vi "Overview of Qs.vi"() -> ()   [LabVIEW 2021, in "Qs.lvlib"]
uses:
  Qs.lvlib
panel:
  in  "Numeric Control":i32
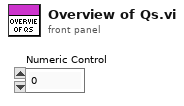
[diagram p1: front panel]
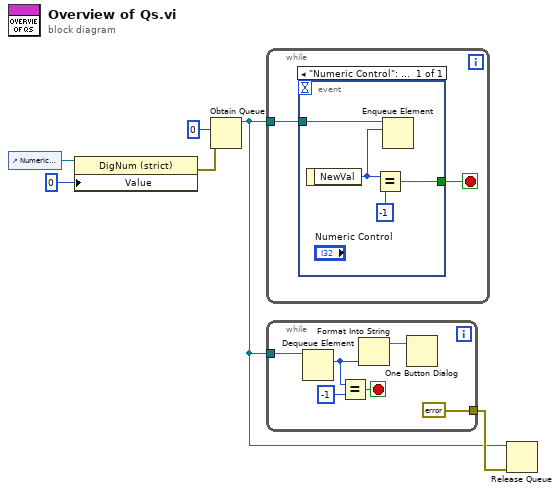
[diagram p0: block diagram]
diagram:
  n1 = control-ref of="Numeric Control"() -> (w6:refnum<vi>)
  n2 = property class="DigNum (strict)"(reference=w6, "Value"=0) -> (error out=w5:errorcluster)  [unwired: 1 in, 1 out]
  n3 = Obtain Queue(element data type=0 ("Value"), error in (no error)=w5) -> (queue out=w1:refnum<queue>)  [unwired: 3 in, 2 out]
  n4 = while {
    tunnel: w1 -> [w7]
    stop <- w8 stop-if-true
    n5 = event shown="[0] \"Numeric Control\": Value Change" {
      selector: _ -> [_]
      dyn-events: _ -> [_]
      timeout: _ -> [_]
      tunnel: w7 -> [w9]
      tunnel: [w11] -> w8
      event "Numeric Control": Value Change {
        n6 = event-data() -> ("NewVal"=w10:i32)  [unwired: 1 in]
        n7 = Equal?(x=w10, y=-1) -> (x = y?=w11:bool)
        n8 = Enqueue Element(queue=w9, element=w10) -> ()  [unwired: 2 in, 3 out]
      }
    }
  }
  n9 = while {
    tunnel: w1 -> [w15]
    tunnel: [errorcluster {"status"=FALSE, "code"=0, "source"=""} ("error in (no error)")] -> w3
    stop <- w18 stop-if-true
    n10 = Dequeue Element(queue=w15) -> (element=w13:i32)  [unwired: 2 in, 3 out]
    n11 = Equal?(x=w13, y=-1) -> (x = y?=w18:bool)
    n12 = Format Into String(w13) -> (resulting string=w14:string)  [unwired: 3 in, 1 out]
    n13 = One Button Dialog(message=w14) -> ()  [unwired: 1 in, 1 out]
  }
  n14 = Release Queue(queue=w1, error in (no error)=w3) -> ()  [unwired: 1 in, 3 out]
